vi "fgv_ctrl-refs.vi"(7 "cmd":T2, 11 "ref":T1) -> (3 "ref 2":T1)   [LabVIEW 2021]
uses:
  ctrl/rw.ctl
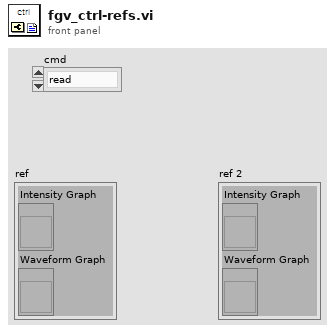
[diagram p1: front panel]
types:
  T1 = cluster{"Intensity Graph":refnum<vi>, "Waveform Graph":refnum<vi>}
  T2 = typedef "rw.ctl" = enum16{"read", "write"}
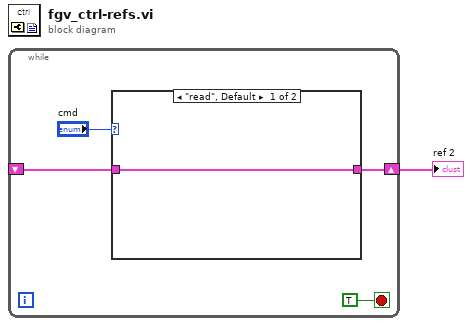
[diagram p0: block diagram]
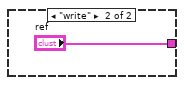
[diagram p2: hidden frame]
diagram:
  n1 = while {
    shift-right: [w3] -> w1
    shift-left: _ -> [w2]
    stop <- TRUE stop-if-true
    n2 = case shown="\"read\", Default" "cmd" {
      tunnel: [w6 "ref"] -> w3
      tunnel: w2 -> [w6 _]
      frame "read", Default {
      }
      frame "write" {
      }
    }
  }
  "ref 2" <- w1
